vi "Cal RHS (Numeric).vi"(8 "error in (no error)":errorcluster, 10 "RHS in":variant, 11 "Domain_Evolut_2D_Rect in":refnum<class "NI_Domain_Evolut_2D_Rect.lvclass">) -> (0 "error out":errorcluster, 2 "RHS out":variant, 3 "Domain_Evolut_2D_Rect out":refnum<class "NI_Domain_Evolut_2D_Rect.lvclass">)   [LabVIEW 2020, in "NI_PDE.lvlib" / "NI_Domain_Evolut_2D_Rect.lvclass"]
uses:
  <vilib>/gmath/pde.llb/DomainClass/Domain_Evolut_2D_Rect/NI_Domain_Evolut_2D_Rect.lvclass
  <vilib>/gmath/pde.llb/DomainClass/Domain_Evolut_2D_Rect/NI_Domain_Evolut_2D_Rect.lvclass/NI_Domain_Evolut_2D_Rect.ctl
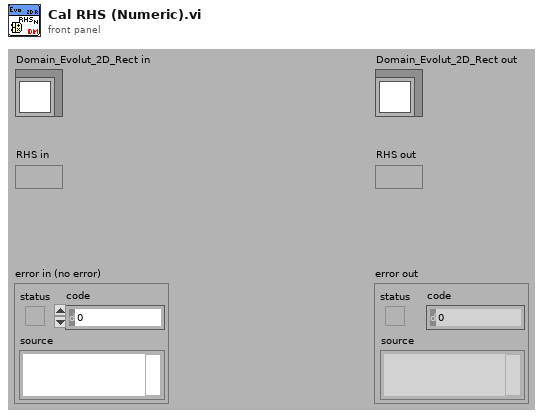
[diagram p1: front panel]
types:
  T1 = cluster{"initial t":dbl, "final t":dbl, "# of t-points":i32}
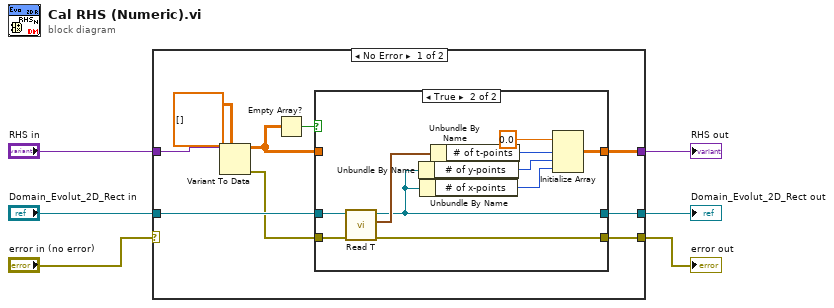
[diagram p0: block diagram]
diagram:
  n1 = case shown="No Error" "error in (no error)" {
    selector: "error in (no error)" -> [_ w31]
    tunnel: "Domain_Evolut_2D_Rect in" -> [w11 w30]
    tunnel: [w7 w30] -> w6
    tunnel: [w8 w31] -> w5
    tunnel: [w9 w29] -> w2
    tunnel: "RHS in" -> [w15 w29]
    frame No Error {
      n2 = Variant To Data(type=dbl[][][] [] ("F"), Variant=w15) -> (data=w12:dbl[][][], error out=w10:errorcluster)  [unwired: 1 in]
      n3 = Empty Array?(array=w12) -> (empty?=w13:bool)
      n4 = case shown="True" w13 {
        tunnel: w11 -> [w16 w23]
        tunnel: w10 -> [w17 w22]
        tunnel: w12 -> [w18 _]
        tunnel: [w17 w28] -> w8
        tunnel: [w18 w25] -> w9
        tunnel: [w16 w19] -> w7
        frame False {
        }
        frame True {
          n5 = call-dynamic "Read T.vi"("error in (no error)"=w22, "Domain_Evolut.lvclass in"=w23) -> ("error out"=w28:errorcluster, "t"=w26:T1, "Domain_Evolut.lvclass out"=w19:refnum<class "NI_Domain_Evolut_2D_Rect.lvclass">)  [unwired: 7 out]
          n6 = Unbundle By Name(w19) -> ("# of y-points"=w21:i32)
          n7 = Unbundle By Name(w19) -> ("# of x-points"=w20:i32)
          n8 = Unbundle By Name(w26) -> ("# of t-points"=w24:i32)
          n9 = Initialize Array(0.0 ("element"), w24, w21, w20) -> (w25:dbl[][][])
        }
      }
    }
    frame Error {
    }
  }
  "Domain_Evolut_2D_Rect out" <- w6
  "error out" <- w5
  "RHS out" <- w2
